vi "Handle Command.vi"(8 "error in":errorcluster, 10 "CMD in":refnum<class "Change Laser Rep Rate CMD.lvclass">, 11 "Object In":refnum<class>) -> (0 "error out":errorcluster, 1 "Command Successful?":bool, 2 "CMD out":refnum<class "Change Laser Rep Rate CMD.lvclass">, 3 "Object Out":refnum<class>)   [LabVIEW 2016, in "gCRDS.lvlib" / "Change Laser Rep Rate CMD.lvclass"]
doc: "This VI will contain the code used to actually execute the request. If the request is successful, this will be indicated by the boolean output <b>Command Successful?</b>. The boolean output can then be used by the <b>Command Reply</b> which sends a reply if the reply queue is valid."
uses:
  Change Laser Rep Rate CMD.lvclass
  <vilib>/MSR Consulting, LLC/General Reuse/Session APIs/Session Log/System Log.lvclass
  gCRD.lvclass
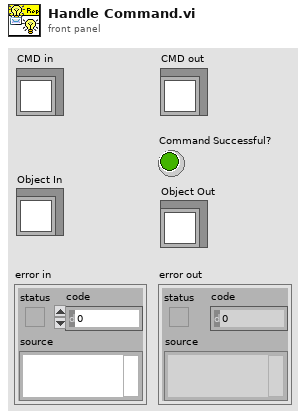
[diagram p1: front panel]
types:
  T1 = typedef "Session - Root.lvclass/Session Handle.ctl" = refnum<data-value>
  T2 = cluster{"tag":string, "section":string, "data":variant}
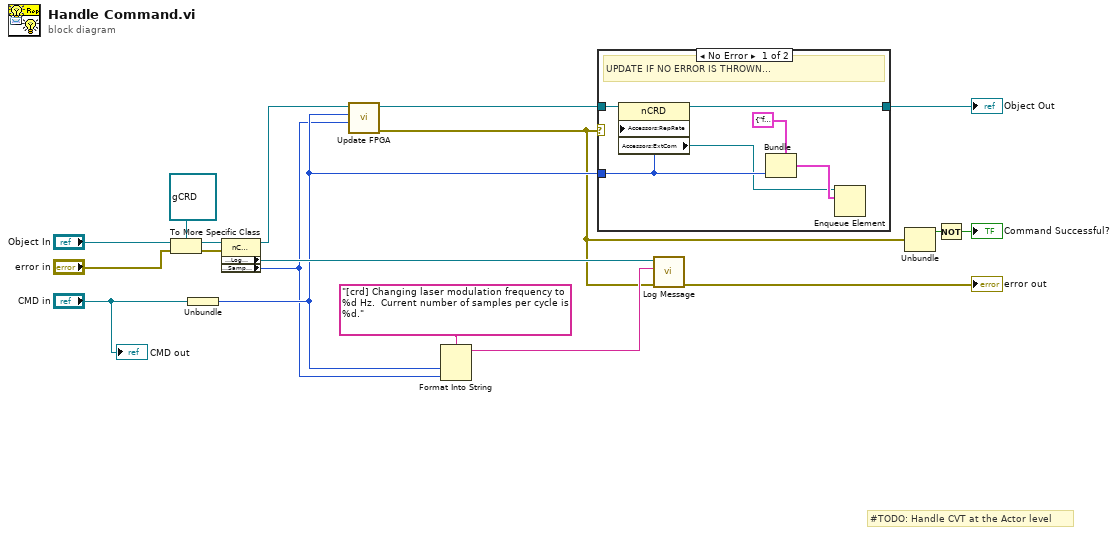
[diagram p0: block diagram]
diagram:
  # "#TODO: Handle CVT at the Actor level"
  n1 = To More Specific Class(target class=refnum<class "gCRD.lvclass"> refnum ("gCRDS.lvlib:nCRD"), reference="Object In", error in="error in") -> (specific class reference=w18:refnum<class "gCRD.lvclass">, error out=w17:errorcluster)
  n2 = Unbundle("CMD in") -> (w3:u16)
  n3 = property class="nCRD"(reference=w18, error in=w17) -> (reference out=w5:refnum<class "gCRD.lvclass">, "Accessors:Log Session"=w16:T1, "Accessors:SamplesPerCycle"=w1:u16)  [unwired: 1 out]
  n4 = call "Update FPGA.vi"("Samples per Cycle"=w1, "RepRate"=w3, "gCRDS"=w5) -> ("error out"=w2:errorcluster, "gCRDS"=w4:refnum<class "gCRD.lvclass">)  [unwired: 7 in]
  n5 = Format Into String(format string="[crd] Changing laser modulation frequency to %d Hz.  Current number of samples per cycle is %d.", w3, w1) -> (resulting string=w14:string)  [unwired: 2 in, 1 out]
  n6 = case shown="No Error" w2 {
    tunnel: w4 -> [w22 w25]
    tunnel: [w21 w25] -> w12
    tunnel: w3 -> [w20 _]
    frame No Error {
      # "UPDATE IF NO ERROR IS THROWN..."
      n7 = property class="nCRD"(reference=w22, "Accessors:RepRate"=w20) -> (reference out=w21:refnum<class "gCRD.lvclass">, "Accessors:ExtCom"=w19:refnum<queue>)  [unwired: 1 in, 1 out]
      n8 = Bundle(cluster=T2 {"tag"="f", "section"="crd", "data"=variant} ("element"), "data"=w20) -> (w23:T2)  [unwired: 2 in]
      n9 = Enqueue Element(queue=w19, element=w23) -> ()  [unwired: 2 in, 3 out]
    }
    frame Error {
    }
  }
  "Object Out" <- w12
  n10 = call <vilib>:"Log Message.vi"("error in"=w2, "MSG In"=w14, "session in"=w16) -> ("error out"=→"error out":errorcluster)  [unwired: 7 in, 1 out]
  n11 = Unbundle(w2) -> ("status"=w7:bool)  [unwired: 2 out]
  n12 = Not(x=w7) -> (.not. x?=→"Command Successful?":bool)
  "CMD out" <- "CMD in"
